vi "Set Text.vi"(8 "Error In":errorcluster, 10 "Text":string, 11 "Label In":refnum<k24>) -> (0 "Error Out":errorcluster, 3 "Label Out":refnum<k24>)   [LabVIEW 2020, in "Dot Net UI Controls.lvlib"]
uses:
  Dot Net UI Controls.lvlib
  System.Windows.Forms
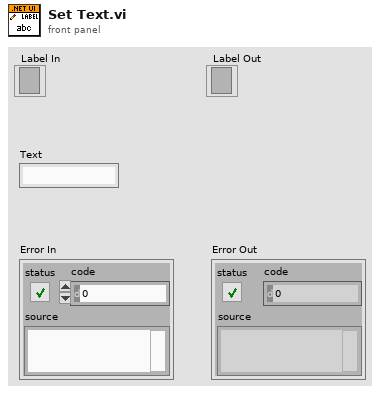
[diagram p1: front panel]
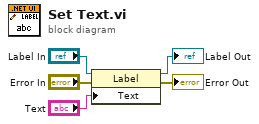
[diagram p0: block diagram]
diagram:
  n1 = property class="Label"(reference="Label In", error in="Error In", "Text"="Text") -> (reference out=→"Label Out":refnum<k24>, error out=→"Error Out":errorcluster)
